vi "Auto Manager.vi"   [LabVIEW 2020]
uses:
  Team Code/Robot Global Data.vi
types:
  T1 = typedef "Auton Cluster Typedef.ctl" = cluster{"rotation":dbl, "maxVelocity(%)":dbl, "delayTime(s)":dbl, "endCondition":dbl, "noSlow":dbl, "intake":dbl, "shooterSpinup":dbl, "shoot":dbl, "X":dbl, "Y":dbl, "maxRotation(%)":dbl, "ballsToShoot":dbl, "ballsToCollect":dbl, "spit":dbl}
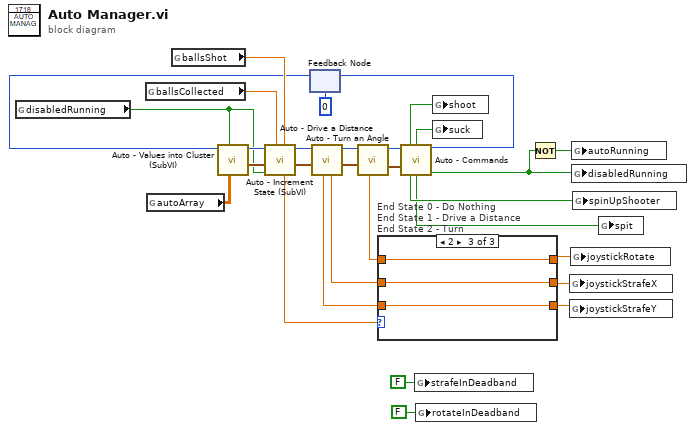
[diagram p0: block diagram]
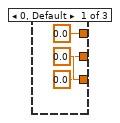
[diagram p2: hidden frame]
diagram:
  n1 = global read "Robot Global Data.vi" "disabledRunning"() -> (w7:bool)
  n2 = global read "Robot Global Data.vi" "ballsCollected"() -> (w6:dbl)
  n3 = global read "Robot Global Data.vi" "autoArray"() -> (w11:dbl[][])
  n4 = global read "Robot Global Data.vi" "ballsShot"() -> (w5:dbl)
  n5 = feedback #1(0 ("Auton State Out")) -> (w3:i32)
  n6 = call "Auto - Values into Cluster (SubVI).vi"("Auto Array"=w11, "Was Disabled"=w7, "Auton State"=w3) -> ("Auton Input Cluster With Data"=w27:T1, "Auton State Out"=w28:i32)  [unwired: 7 in]
  n7 = call "Auto - Increment State (SubVI).vi"("ballsShot"=w5, "ballsCollected"=w6, "disabledRunning"=w7, "Auton Cluster In"=w27, "Auton State In"=w28) -> ("Auton cluster Out"=w26:T1, "Auton State Out"=w17:i32, "End Condition"=w24:dbl)  [unwired: 4 in]
  n8 = call "Auto - Drive a Distance.vi"("Auton Cluster In"=w26, "Auton State In"=w17) -> ("Auton Cluster Out"=w25:T1, "Auton State Out"=w16:i32, "Strafe Y (ROBOT)"=w22:dbl, "Strafe X (ROBOT)"=w23:dbl)  [unwired: 6 in]
  n9 = call "Auto - Turn an Angle.vi"("Auton Cluster In"=w25, "Auton State In"=w16) -> ("Auton Cluster Out"=w14:T1, "Auton State Out"=w15:i32, "rotation"=w19:dbl)  [unwired: 7 in]
  n10 = case "End State 0 - Do Nothing\nEnd State 1 - Drive a Distance\nEnd State 2 - Turn" shown="2" w24 {
    tunnel: w23 -> [_ w34 w37]
    tunnel: w22 -> [_ w35 w38]
    tunnel: [0.0 ("Strafe Y (ROBOT)") w34 w37] -> w20
    tunnel: [0.0 ("Strafe X (ROBOT)") w35 w38] -> w21
    tunnel: w19 -> [_ w36 w39]
    tunnel: [0.0 ("rotation") w36 w39] -> w18
    frame 0, Default {
    }
    frame 1 {
    }
    frame 2 {
    }
  }
  n11 = call "Auto - Commands.vi"("Auton State In"=w15, "Auton Cluster In"=w14) -> ("shoot"=w13:bool, "suck"=w12:bool, "Auton State Out"=w4:i32, "shooterSpinup"=w2:bool, "spit"=w1:bool, "disabledRunning"=w9:bool)  [unwired: 7 in, 1 out]
  n12 = feedback-in #1(w4) -> ()
  n13 = global write "Robot Global Data.vi" "strafeInDeadband"(FALSE ("strafeInDeadband")) -> ()
  n14 = global write "Robot Global Data.vi" "rotateInDeadband"(FALSE ("rotateInDeadband")) -> ()
  n15 = global write "Robot Global Data.vi" "shoot"(w13) -> ()
  n16 = global write "Robot Global Data.vi" "suck"(w12) -> ()
  n17 = Not(x=w9) -> (.not. x?=w8:bool)
  n18 = global write "Robot Global Data.vi" "joystickStrafeX"(w21) -> ()
  n19 = global write "Robot Global Data.vi" "joystickStrafeY"(w20) -> ()
  n20 = global write "Robot Global Data.vi" "joystickRotate"(w18) -> ()
  n21 = global write "Robot Global Data.vi" "autoRunning"(w8) -> ()
  n22 = global write "Robot Global Data.vi" "disabledRunning"(w9) -> ()
  n23 = global write "Robot Global Data.vi" "spinUpShooter"(w2) -> ()
  n24 = global write "Robot Global Data.vi" "spit"(w1) -> ()
